vi "Close.vi"(8 "error in (no error)":errorcluster, 11 "Masterflex Settings in":T1={"VISA resource name"="", "Simulated?"=FALSE, "Pump Number"=1.0, "Reverse?"=FALSE} {"Pump Number" min=1.0 max=20.0 step=1.0}) -> (0 "error out":errorcluster, 1 "Connection Error":bool, 3 "Masterflex Settings out":T1={"VISA resource name"="", "Simulated?"=FALSE, "Pump Number"=1.0, "Reverse?"=FALSE} {"Pump Number" min=1.0 max=20.0 step=1.0})   [LabVIEW 2018, in "Masterflex 7550-30.lvlib"]
uses:
  Masterflex 7550-30.lvlib
  Controls/Settings Cluster.ctl
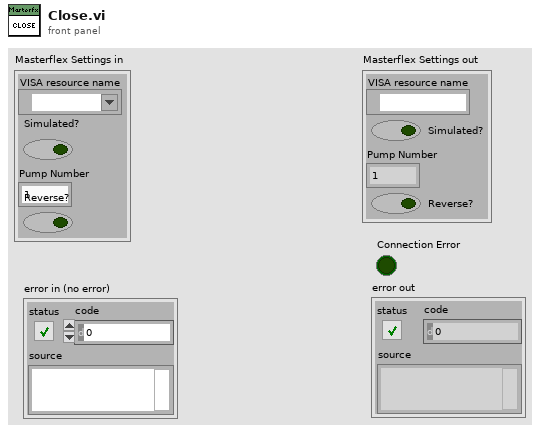
[diagram p1: front panel]
types:
  T1 = typedef "Masterflex 7550-30.lvlib/Settings Cluster.ctl" = cluster{"VISA resource name":refnum<visa-resource-name>, "Simulated?":bool, "Pump Number":dbl, "Reverse?":bool}
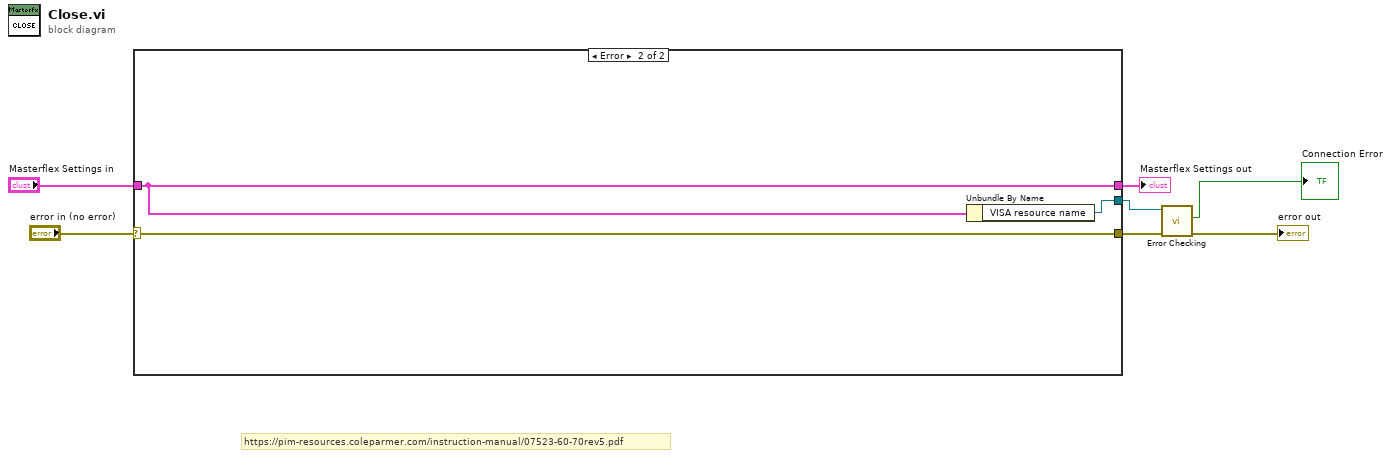
[diagram p0: block diagram]
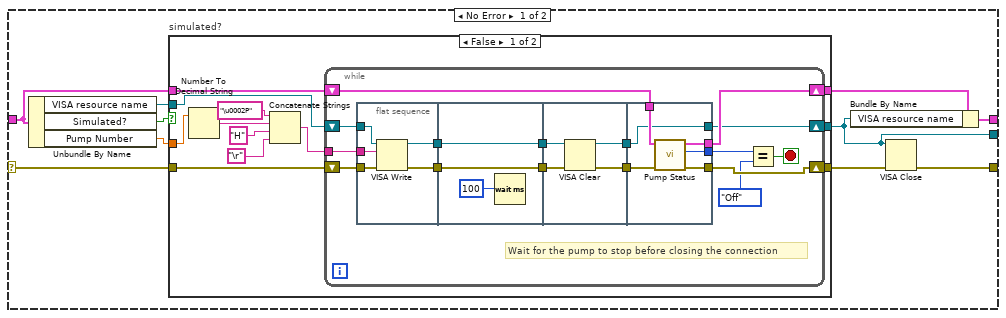
[diagram p2: hidden frame]
diagram:
  # "https://pim-resources.coleparmer.com/instruction-manual/07523-60-70rev5.pdf"
  n1 = case shown="Error" "error in (no error)" {
    selector: "error in (no error)" -> [w14 w69]
    tunnel: [w9 w69] -> w2
    tunnel: [w16 w68] -> w5
    tunnel: "Masterflex Settings in" -> [w12 w68]
    tunnel: [w8 w67] -> w3
    frame No Error {
      n2 = Unbundle By Name(w12) -> ("VISA resource name"=w13:refnum<visa-resource-name>, "Simulated?"=w17:bool, "Pump Number"=w15:dbl)
      n3 = case "simulated?" shown="False" w17 {
        tunnel: [w29 w65] -> w10
        tunnel: [w19 w64] -> w8
        tunnel: w15 -> [w25 _]
        tunnel: w14 -> [w23 w65]
        tunnel: w13 -> [w18 w64]
        tunnel: w12 -> [w21 w66]
        tunnel: [w20 w66] -> w11
        frame False {
          n4 = Number To Decimal String(number=w25) -> (decimal integer string=w24:string)  [unwired: 1 in]
          n5 = Concatenate Strings("\u0002P" ("string"), w24, "H" ("string"), "\r") -> (w22:string)
          n6 = while {
            tunnel: w22 -> [w38]
            shift-right: [w40] -> w29
            shift-left: w23 -> [w39]
            shift-right: [w36] -> w20
            shift-left: w21 -> [w37]
            shift-right: [w35] -> w19
            shift-left: w18 -> [w33]
            stop <- w31 stop-if-true
            # "Wait for the pump to stop before closing the connection"
            n7 = flat-sequence {
              tunnel: [w46] -> w45
              tunnel: [w47] -> w44
              tunnel: w39 -> [w50]
              tunnel: w38 -> [w49]
              tunnel: w33 -> [w48]
              tunnel: [w53] -> w43
              tunnel: [w52] -> w42
              tunnel: w45 -> [w53]
              tunnel: w44 -> [w52]
              tunnel: w43 -> [w57]
              tunnel: w42 -> [w56]
              tunnel: [w55] -> w41
              tunnel: [w54] -> w34
              tunnel: [w62] -> w40
              tunnel: w41 -> [w63]
              tunnel: w37 -> [w61]
              tunnel: [w60] -> w36
              tunnel: [w59] -> w32
              tunnel: [w58] -> w35
              tunnel: w34 -> [w58]
              frame #0 {
                n8 = VISA Write(VISA resource name=w48, write buffer=w49, error in (no error)=w50) -> (VISA resource name out=w46:refnum<visa-resource-name>, error out=w47:errorcluster)  [unwired: 1 out]
              }
              frame #1 {
                n9 = Wait (ms)(milliseconds to wait=u32 100) -> ()  [unwired: 1 out]
              }
              frame #2 {
                n10 = VISA Clear(VISA resource name=w57, error in (no error)=w56) -> (VISA resource name out=w54:refnum<visa-resource-name>, error out=w55:errorcluster)
              }
              frame #3 {
                n11 = call "Pump Status.vi"("error in (no error)"=w63, "Masterflex Settings in"=w61) -> ("error out"=w62:errorcluster, "Pump On?"=w59:enum16{"Off", "On", "Not Initialized"}, "Masterflex Settings out"=w60:T1)  [unwired: 6 in, 1 out]
              }
            }
            n12 = Equal?(x=w32, y=enum16{"Off", "On", "Not Initialized"}."Off") -> (x = y?=w31:bool)
          }
        }
        frame True {
        }
      }
      n13 = Bundle By Name(cluster=w11, "VISA resource name"=w8) -> (w16:T1)
      n14 = VISA Close(VISA resource name=w8, error in (no error)=w10) -> (error out=w9:errorcluster)
    }
    frame Error {
      n15 = Unbundle By Name(w68) -> ("VISA resource name"=w67:refnum<visa-resource-name>)
    }
  }
  "Masterflex Settings out" <- w5
  n16 = call "Error Checking.vi"("error in (no error)"=w2, "VISA resource name"=w3) -> ("error out"=→"error out":errorcluster, "Connection Error"=→"Connection Error":bool)  [unwired: 7 in, 1 out]
